vi "View Distance Write.vi"(8 "error in (no error)":errorcluster, 9 "Distance":sgl, 11 "3D Plot.lvclass in":refnum<class "3D Plot.lvclass">) -> (0 "error out":errorcluster, 3 "3D Plot.lvclass out":refnum<class "3D Plot.lvclass">)   [LabVIEW 2017, in "3D Plot.lvclass"]
uses:
  <vilib>/Math Plots/3D Math Plots/3D Plot/3D Plot/3D Plot.lvclass
  <vilib>/Math Plots/3D Math Plots/3D Plot/3D Plot/3D Plot.lvclass/3D Plot.ctl
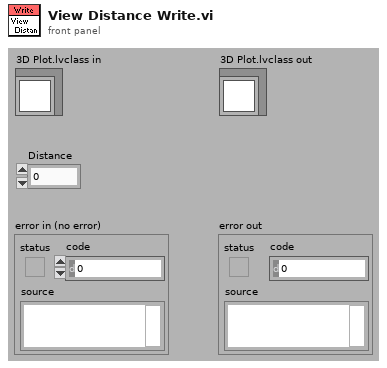
[diagram p1: front panel]
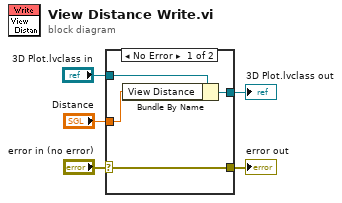
[diagram p0: block diagram]
diagram:
  n1 = case shown="No Error" "error in (no error)" {
    selector: "error in (no error)" -> [w6 w10]
    tunnel: "Distance" -> [w9 _]
    tunnel: "3D Plot.lvclass in" -> [w8 w11]
    tunnel: [w7 w11] -> w3
    tunnel: [w6 w10] -> w1
    frame No Error {
      n2 = Bundle By Name(cluster=w8, "View Distance"=w9) -> (w7:refnum<class "3D Plot.lvclass">)
    }
    frame Error {
    }
  }
  "3D Plot.lvclass out" <- w3
  "error out" <- w1
